vi "tarea.vi"() -> ()   [LabVIEW 2011]
panel:
  out "Sobresalientes":bool
  out "Muy buenos":bool
  out "Reprobados":bool
  out "Buenos":bool
  out "Sobresalientes":dbl
  out "Muy buenos":dbl
  out "Buenos":dbl
  out "Reprobados":dbl
  # "Generar la nota de 10 alumnos, luego ir contando cuantos alumnos estan en los siguientes rangos\n\n1-59 reprobados\n60-80 buenos\n81-90 muy buenos\n91-100 sobresalientes\n\nEncender un led para cada uno de los rangos."
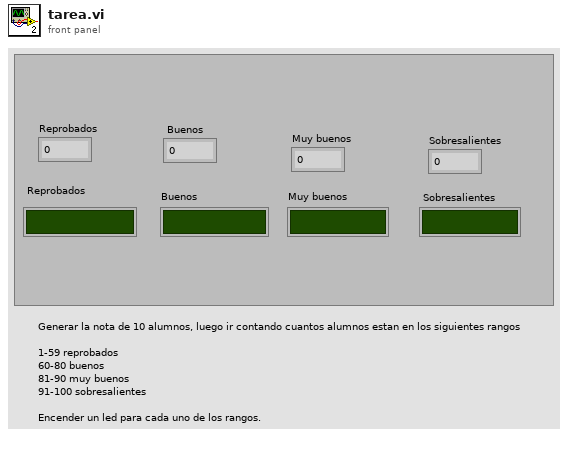
[diagram p1: front panel]
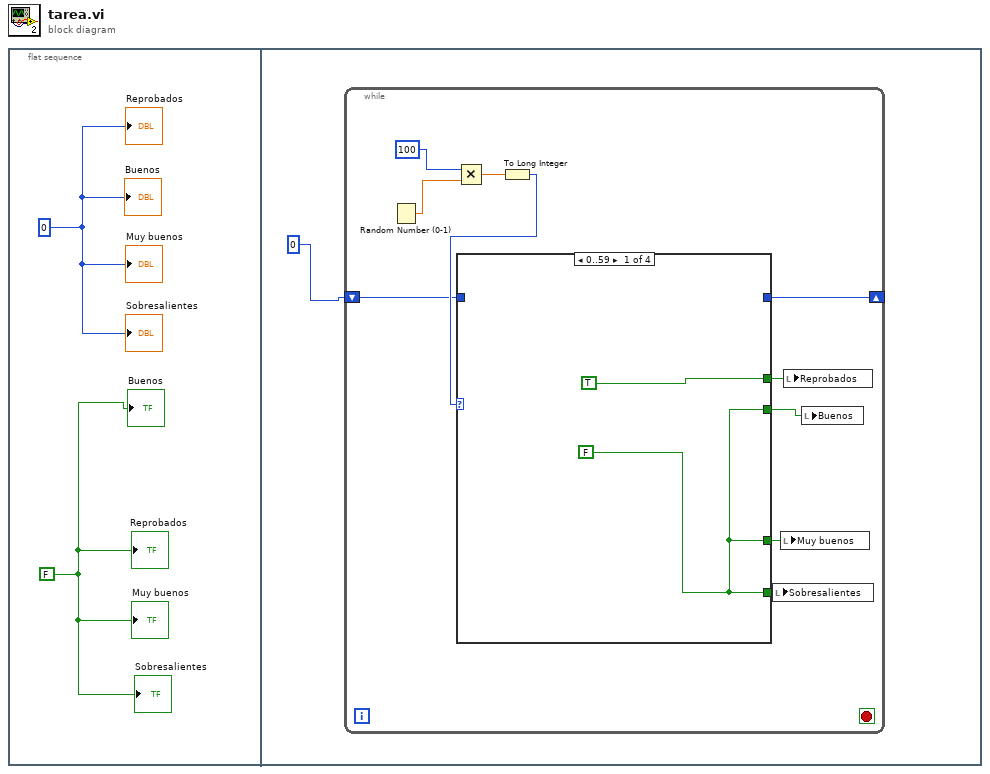
[diagram p0: block diagram]
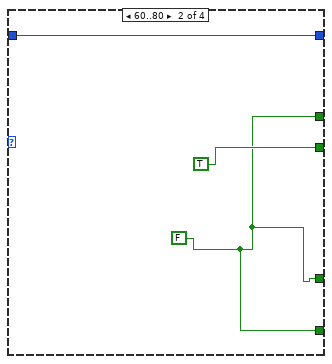
[diagram p2: hidden frame]
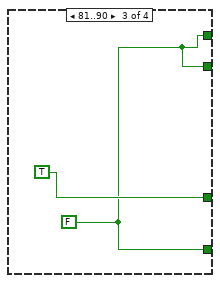
[diagram p3: hidden frame]
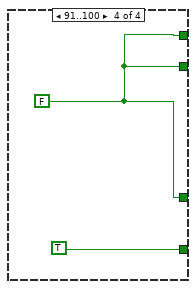
[diagram p4: hidden frame]
diagram:
  n1 = flat-sequence {
    frame #0 {
      w2 = FALSE
      w1 = 0
      "Reprobados" <- w1
      "Buenos" <- w1
      "Muy buenos" <- w1
      "Sobresalientes" <- w1
      "Buenos" <- w2
      "Reprobados" <- w2
      "Muy buenos" <- w2
      "Sobresalientes" <- w2
    }
    frame #1 {
      n2 = while {
        shift-right: [w8] -> _
        shift-left: 0 -> [w9]
        stop <- _ stop-if-true
        n3 = Random Number (0-1)() -> (number: 0 to 1=w12:dbl)
        n4 = Multiply(x=100, y=w12) -> (x*y=w11:dbl)
        n5 = To Long Integer(number=w11) -> (32bit integer=w10:i32)
        n6 = case shown="0..59" w10 {
          tunnel: [_ w16 _ _] -> w8
          tunnel: w9 -> [_ w16 _ _]
          tunnel: [w15 w17 w19 TRUE] -> w7
          tunnel: [w15 TRUE w19 w22] -> w6
          tunnel: [w15 w17 TRUE w22] -> w5
          tunnel: [TRUE w17 w19 w22] -> w4
          frame 0..59 {
            w15 = FALSE
          }
          frame 60..80 {
            w17 = FALSE
          }
          frame 81..90 {
            w19 = FALSE
          }
          frame 91..100 {
            w22 = FALSE
          }
        }
        n7 = local write "Sobresalientes"(w7) -> ()
        n8 = local write "Muy buenos"(w5) -> ()
        n9 = local write "Reprobados"(w4) -> ()
        n10 = local write "Buenos"(w6) -> ()
      }
    }
  }
